vi "Color Wheel Command Handler.vi"(6 "Operator POVs":i16[](array[numeric]), 7 "Driver POVs":i16[](array[numeric]), 8 "Operator Axes":dbl[](array[numeric]), 9 "Operator Buttons":bool[](array[boolean]), 10 "Driver Buttons":bool[](array[boolean]), 11 "Driver Axes":dbl[](array[numeric])) -> ()   [LabVIEW 2019]
uses:
  c0e63fae-867d-4df3-95cf-ee7c9b7e9c6d.vi
  7b3b5119-3f72-42ea-99e4-d46ebab760ea.vi
  <vilib>/Rock Robotics/Network Tables/NT Write Number.vi
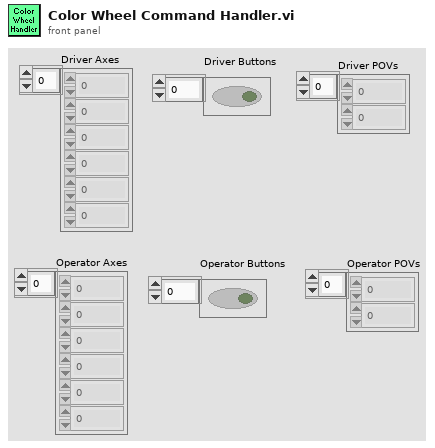
[diagram p1: front panel]
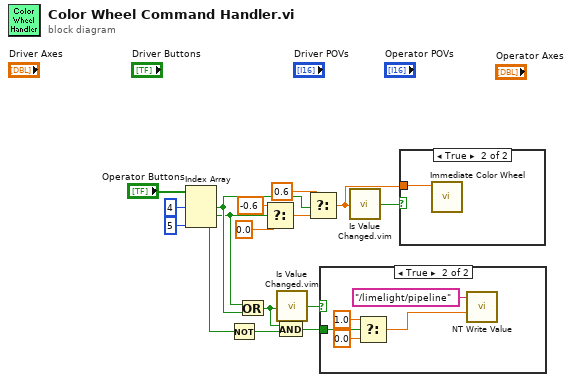
[diagram p0: block diagram]
diagram:
  n1 = Index Array(array="Operator Buttons", index #1=4 ("index"), index #2=5 ("index")) -> (element #1=w7:bool, element #2=w6:bool, element #3=w4:bool)  [unwired: 1 in]
  n2 = Not(x=w4) -> (.not. x?=w3:bool)
  n3 = Or(x=w6, y=w7) -> (x .or. y?=w2:bool)
  n4 = Select(t=-0.6, s=w6, f=0.0) -> (s? t:f=w13:dbl)
  n5 = And(x=w2, y=w3) -> (x .and. y?=w1:bool)
  n6 = call "Is Value Changed.vim"("value"=w2) -> ("changed or first call?"=w5:bool)
  n7 = Select(t=0.6, s=w7, f=w13) -> (s? t:f=w8:dbl)
  n8 = case shown="True" w5 {
    tunnel: w1 -> [_ w20]
    frame False {
    }
    frame True {
      n9 = Select(t=1.0, s=w20, f=0.0) -> (s? t:f=w17:dbl)
      n10 = call-poly <vilib>:"NT Write Value.vi"("Numeric"=w17, "Name"="/limelight/pipeline") -> ()  [unwired: 9 in, 1 out]
    }
  }
  n11 = call "Is Value Changed.vim"("value"=w8) -> ("changed or first call?"=w9:bool)
  n12 = case shown="True" w9 {
    tunnel: w8 -> [_ w22]
    frame False {
    }
    frame True {
      n13 = call "Immediate Color Wheel.vi"("Setpoint"=w22) -> ()  [unwired: 11 in]
    }
  }
